vi "Empty Specific Notifier.vi"(8 "error in (no error)":errorcluster, 10 "ID In":variant, 11 "Simple Map SEQ I64 Notifier Controller in":refnum<class "Simple Map SEQ I64 Notifier Controller.lvclass">) -> (0 "error out":errorcluster, 3 "Simple Map SEQ I64 Notifier Controller out":refnum<class "Simple Map SEQ I64 Notifier Controller.lvclass">)   [LabVIEW 2019, in "Simple Map SEQ I64 Notifier Controller.lvclass"]
uses:
  Simple Map SEQ I64 Notifier Controller.lvclass
  Simple Map SEQ I64 Notifier Controller.lvclass/Simple Map SEQ I64 Notifier Controller.ctl
  Ancestor Class/Actor Assistant/Notifier/Notifier.lvclass
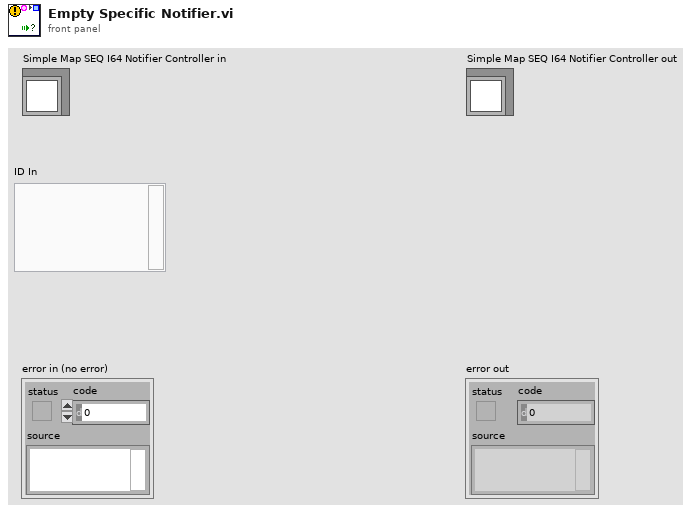
[diagram p1: front panel]
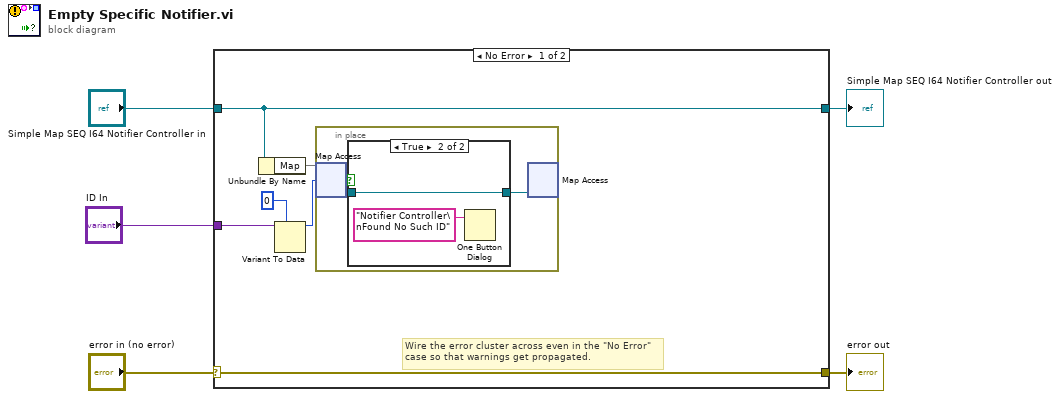
[diagram p0: block diagram]
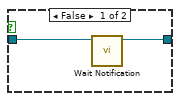
[diagram p2: hidden frame]
diagram:
  n1 = case shown="No Error" "error in (no error)" {
    selector: "error in (no error)" -> [w11 w20]
    tunnel: [w11 w20] -> w4
    tunnel: [w9 w19] -> w2
    tunnel: "Simple Map SEQ I64 Notifier Controller in" -> [w9 w19]
    tunnel: "ID In" -> [w10 _]
    frame No Error {
      # "Wire the error cluster across even in the \"No Error\"\ncase so that warnings get propagated."
      n2 = Unbundle By Name(w9) -> ("Map"=w8:map{i64, refnum<class "Notifier.lvclass">})
      n3 = Variant To Data(type=i64 0, Variant=w10) -> (data=w6:i64)  [unwired: 1 in, 1 out]
      n4 = in-place {
        n5 = in-place-map #1(w8, w6) -> (w14:refnum<class "Notifier.lvclass">, w12:bool)  [unwired: 1 in]
        n6 = case shown="True" w12 {
          tunnel: w14 -> [w16 w18]
          tunnel: [w15 w18] -> w13
          frame False {
            n7 = call-dynamic "Wait Notification.vi"("Notifier in"=w16) -> ("Notifier out"=w15:refnum<class "Notifier.lvclass">)  [unwired: 7 in, 3 out]
          }
          frame True {
            n8 = One Button Dialog(message="Notifier Controller\nFound No Such ID") -> ()  [unwired: 1 in, 1 out]
          }
        }
        n9 = in-place-map #1(w13) -> ()  [unwired: 1 in, 3 out]
      }
    }
    frame Error {
    }
  }
  "error out" <- w4
  "Simple Map SEQ I64 Notifier Controller out" <- w2
